vi "Simulation Main.vi"() -> ()   [LabVIEW 2015]
uses:
  <vilib>/picture/3D Picture Control/Object/Create Object (name).vi
  <vilib>/picture/3D Picture Control/NI_3D Picture Control.lvlib
panel:
  in  "Stop":bool
  in  "About this VI":bool
  in  "Angle 3":dbl(knob) scale=-85.0..85.0
  in  "Angle 2":dbl(knob) scale=-85.0..85.0
  in  "Angle 1":dbl(knob) scale=-85.0..85.0
  out "Robotic Arm Simulation":refnum<vi>(3d-picture)
  # "myRoboLab"
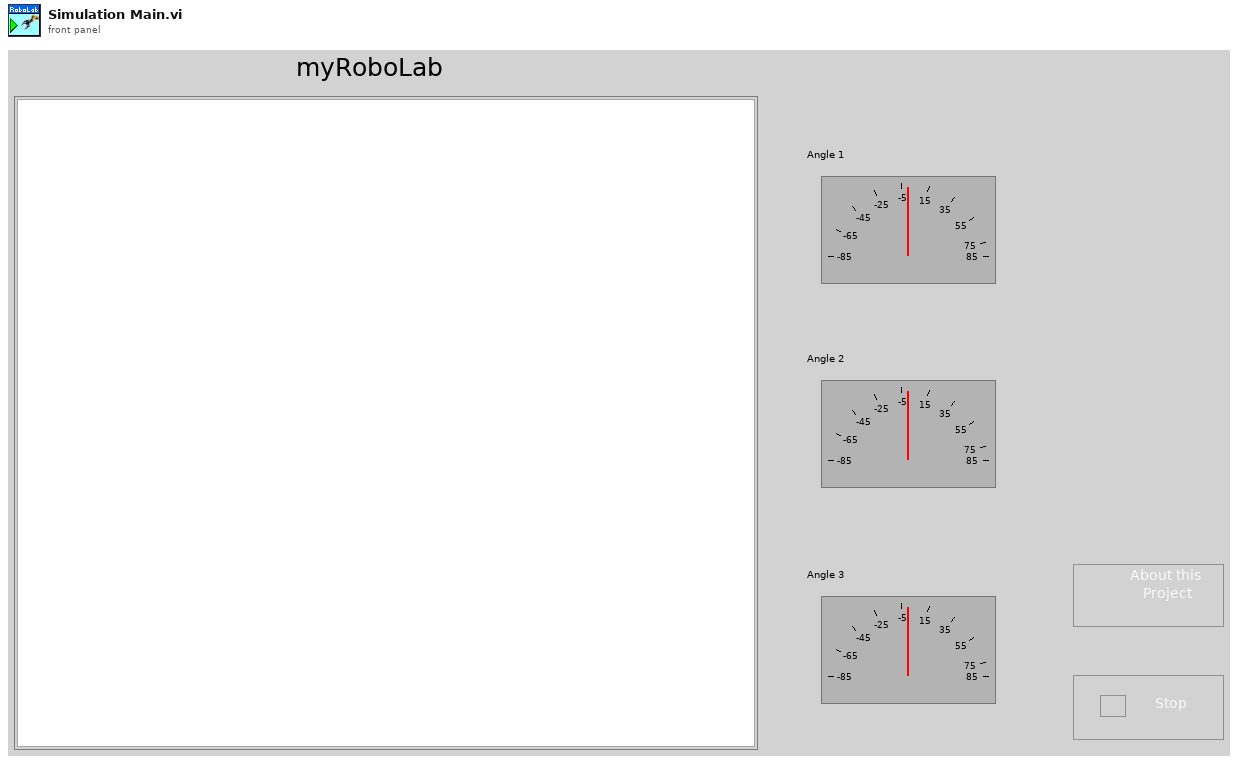
[diagram p1: front panel]
types:
  T1 = cluster{"Red":sgl, "Green":sgl, "Blue":sgl, "Alpha":sgl}
  T2 = typedef "Robotic Parts.ctl" = cluster{"Name":string, "Parent":string, "Type":T3, "Visible?":bool, "Geometry Definition":dbl[], "Position WRT Parent (X,Y,Z)":dbl[], "Rotation WRT Parent (degrees)":dbl[], "Joint Type":T4, "Geometry File Path":path, "Indent Level":i32, "Color":u32}
  T3 = typedef "NI_Robotics_3DKinematics.lvlib/Element Type.ctl" = enum16{"Joint", "Box", "Cylinder", "Cone", "Sphere", "ASE File", "VRML File", "STL File", "Space"}
  T4 = typedef "NI_Robotics_3DKinematics.lvlib/Joint Type.ctl" = enum16{"Trans_X", "Trans_Y", "Trans_Z", "Rot_X", "Rot_Y", "Rot_Z", "None"}
  T5 = typedef "NI_Robotics_3DKinematics.lvlib/Joint Control.ctl" = cluster{"Joint Refnum":refnum<vi>, "Joint Type":T4, "Position WRT Parent":dbl[], "Rotation WRT Parent":dbl[], "Bar Refnum":refnum<vi>}
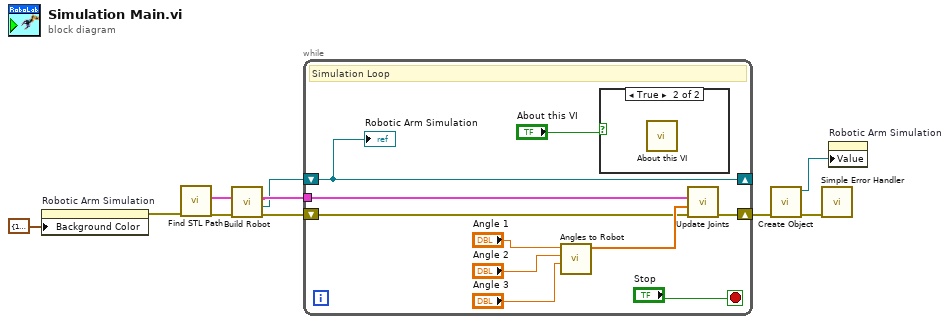
[diagram p0: block diagram]
diagram:
  n1 = property on="Robotic Arm Simulation" class="SceneGraphDisp (strict)"("Background Color"=T1 {"Red"=1.0, "Green"=1.0, "Blue"=1.0, "Alpha"=1.0}) -> (error out=w10:errorcluster)  [unwired: 2 in, 1 out]
  n2 = call "Find STL Path.vi"("Error In"=w10) -> ("Error Out"=w8:errorcluster, "Array for myRoboLab Parts"=w7:T2[])  [unwired: 9 in]
  n3 = call "Build Robot.vi"("error in"=w8, "Robotic Parts"=w7) -> ("error out"=w5:errorcluster, "Scene Out"=w4:refnum<vi>, "Joint Array"=w6:T5[])  [unwired: 7 in]
  n4 = while {
    tunnel: w6 -> [w17]
    shift-right: [w15] -> _
    shift-left: w4 -> [w15]
    shift-right: [w12] -> w3
    shift-left: w5 -> [w16]
    stop <- "Stop" stop-if-true
    # "Simulation Loop"
    n5 = call "Angles to Robot.vi"("Joint 2"="Angle 3", "Joint 1"="Angle 2", "Joint 0"="Angle 1") -> ("Angle array radians"=w20:dbl[])  [unwired: 7 in, 1 out]
    n6 = case shown="True" "About this VI" {
      frame False {
      }
      frame True {
        n7 = call "About this VI.vi"() -> ()  [unwired: 11 in, 1 out]
      }
    }
    n8 = call "Update Joints.vi"("error in (no error)"=w16, "Joints"=w20, "Joint Array"=w17) -> ("error out"=w12:errorcluster)  [unwired: 8 in]
    "Robotic Arm Simulation" <- w15
  }
  n9 = call-poly <vilib>:"Create Object.vi"("error in (no error)"=w3) -> ("error out"=w2:errorcluster, "Scene:New Object"=w1:refnum<vi>)  [unwired: 9 in]
  n10 = call <vilib>:"Simple Error Handler.vi"("error in (no error)"=w2) -> ()  [unwired: 4 in, 5 out]
  n11 = property on="Robotic Arm Simulation" class="SceneGraphDisp (strict)"("Value"=w1) -> ()  [unwired: 2 in, 2 out]
